vi "GetType.vi"(8 "error in (no error)":errorcluster, 11 "Configure Ref Clock Source Msg":refnum<class "Configure Ref Clock Source Msg.lvclass">) -> (0 "error out":errorcluster, 2 "Data Sample":variant, 3 "Configure Ref Clock Source Msg":refnum<class "Configure Ref Clock Source Msg.lvclass">)   [LabVIEW 2015, in "CS++Fgen.lvlib" / "Configure Ref Clock Source Msg.lvclass"]
doc: "This VI delivers a sample of the data type format the message expects."
uses:
  Configure Ref Clock Source Msg.lvclass
  Configure Ref Clock Source Msg.lvclass/Configure Ref Clock Source Msg.ctl
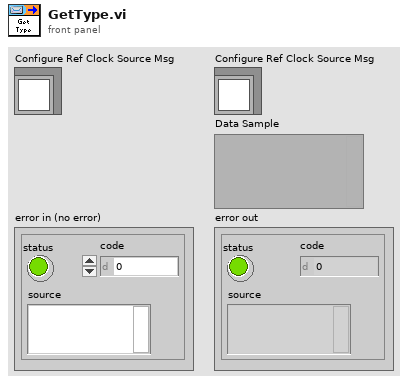
[diagram p1: front panel]
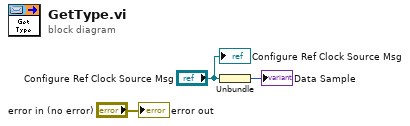
[diagram p0: block diagram]
diagram:
  n1 = Unbundle("Configure Ref Clock Source Msg") -> (→"Data Sample":i32)
  "error out" <- "error in (no error)"
  "Configure Ref Clock Source Msg" <- "Configure Ref Clock Source Msg"
